vi "Refresh Target Information.vi"(7 "Reduce Discovery Timeout":bool=TRUE, 8 "error in (no error)":errorcluster, 10 "User Added Targets Only":bool, 11 "User Added Targets":string[](array[string])) -> (0 "error out":errorcluster, 3 "Targets Information":T1[](array[typedef]) {"Primary NIC"."IP Address Request Mode" items=["Static"=1, "DHCP/Link-Local"=2, "Link-Local Only"=4, "DHCP Only"=8]})   [LabVIEW 2020]
uses:
  Controls/Target Information.ctl
  Controls/Target Network Settings.ctl
  Controls/System Credentials.ctl
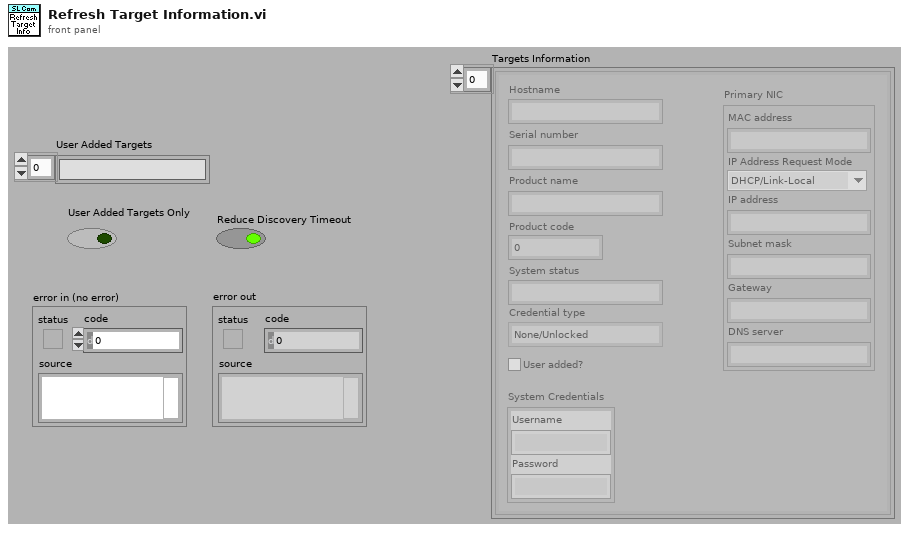
[diagram p1: front panel]
types:
  T1 = typedef "Target Information.ctl" = cluster{"Hostname":string, "Serial number":string, "Product name":string, "Product code":i32, "System status":string, "Credential type":enum16{"None/Unlocked", "FTP Password", "NIAuth Credentials"}, "User added?":bool, "Primary NIC":T2, "System Credentials":T3}
  T2 = typedef "Target Network Settings.ctl" = cluster{"MAC address":string, "IP Address Request Mode":i32, "IP address":string, "Subnet mask":string, "Gateway":string, "DNS server":string}
  T3 = typedef "System Credentials.ctl" = cluster{"Username":string, "Password":string}
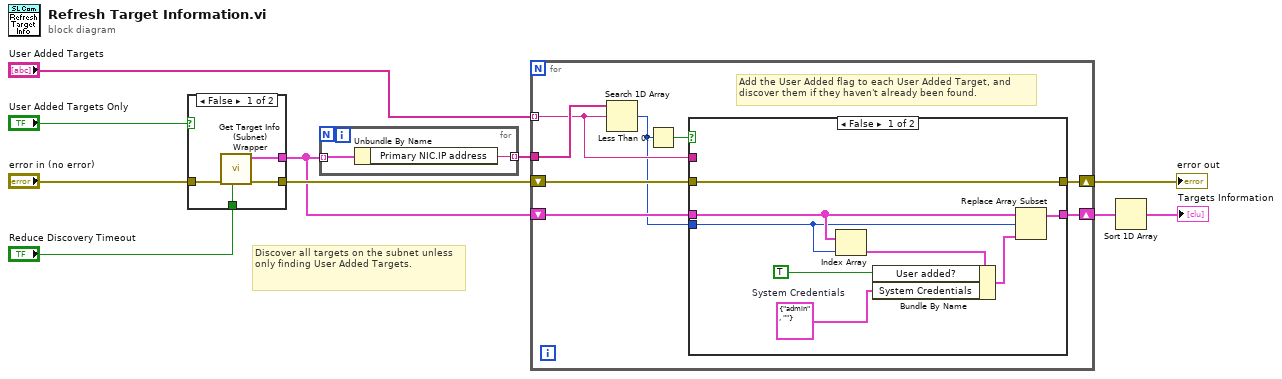
[diagram p0: block diagram]
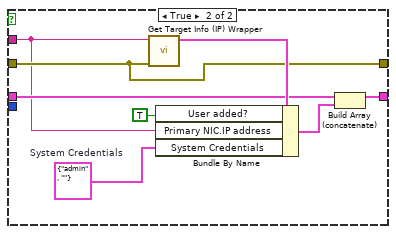
[diagram p2: hidden frame]
diagram:
  # "Discover all targets on the subnet unless only finding User Added Targets."
  n1 = case shown="False" "User Added Targets Only" {
    tunnel: "error in (no error)" -> [w14 w15]
    tunnel: [w13 _] -> w5
    tunnel: [w12 w15] -> w8
    tunnel: "Reduce Discovery Timeout" -> [w11 _]
    frame False {
      n2 = call "Get Target Info (Subnet) Wrapper.vi"("reduce discovery timeout (T)"=w11, "error in (no error)"=w14) -> ("error out"=w12:errorcluster, "target information"=w13:T1[])  [unwired: 8 in]
    }
    frame True {
    }
  }
  n3 = for {
    tunnel: w5 -> [w17] mode=indexing
    tunnel: [w16] -> w6 mode=indexing
    n4 = Unbundle By Name(w17) -> ("Primary NIC.IP address"=w16:string)
  }
  n5 = for {
    tunnel: "User Added Targets" -> [w22] mode=indexing
    tunnel: w6 -> [w24]
    shift-right: [w19] -> w4
    shift-left: w5 -> [w21]
    shift-right: [w18] -> w3
    shift-left: w8 -> [w25]
    # "Add the User Added flag to each User Added Target, and discover them if they haven't already been found."
    n6 = Search 1D Array(1D array=w24, element=w22) -> (index of element=w20:i32)  [unwired: 1 in]
    n7 = Less Than 0?(x=w20) -> (x < 0?=w23:bool)
    n8 = case shown="False" w23 {
      tunnel: w25 -> [w33 w36]
      tunnel: w22 -> [_ w35]
      tunnel: [w33 w36] -> w18
      tunnel: w21 -> [w30 w38]
      tunnel: w20 -> [w27 _]
      tunnel: [w29 w37] -> w19
      frame False {
        w26 = T3 {"Username"="admin", "Password"=""}  # System Credentials
        n9 = Index Array(array=w30, index=w27) -> (element=w32:T1)
        n10 = Bundle By Name(cluster=w32, "User added?"=TRUE ("User Added?"), "System Credentials"=w26) -> (w28:T1)
        n11 = Replace Array Subset(array=w30, new element=w28, index=w27) -> (w29:T1[])
      }
      frame True {
        w34 = T3 {"Username"="admin", "Password"=""}  # System Credentials
        n12 = call "Get Target Info (IP) Wrapper.vi"("error in (no error)"=w36, "target address"=w35) -> ("Target settings"=w41:T1)  [unwired: 8 in, 1 out]
        n13 = Bundle By Name(cluster=w41, "User added?"=TRUE ("User Added?"), "Primary NIC.IP address"=w35, "System Credentials"=w34) -> (w39:T1)
        n14 = Build Array (concatenate)(w38, w39) -> (w37:T1[])
      }
    }
  }
  "error out" <- w3
  n15 = Sort 1D Array(array=w4) -> (sorted array=→"Targets Information":T1[])
